vi "test14-MappingRelationshipByExternalRegistration_State.vi"() -> ()   [LabVIEW 2017, in "testcase-CSMStatusStateRegisterUnregister.lvclass"]
uses:
  testcase-CSMStatusStateRegisterUnregister.lvclass
  src/user.lib/_NEVSTOP/Communicable State Machine(CSM)/AdvanceAPI/CSM - Revert Arguments-Safe String.vi
  src/user.lib/_NEVSTOP/Communicable State Machine(CSM)/AdvanceAPI/CSM - Make String Arguments Safe.vi
  src/user.lib/_NEVSTOP/Communicable State Machine(CSM)/AdvanceAPI/CSM - Break Down Multiple States String.vi
  src/user.lib/_NEVSTOP/Communicable State Machine(CSM)/AdvanceAPI/CSM - Compact Multiple States.vi
  src/user.lib/_NEVSTOP/Communicable State Machine(CSM)/AdvanceAPI/CSM - Keywords.vi
  src/user.lib/_NEVSTOP/Communicable State Machine(CSM)/_Polymophic/CSM - Replace Marks in Messages.vi
  src/user.lib/_NEVSTOP/Communicable State Machine(CSM)/_Shared/Trim Single-line Text.vi
  src/user.lib/_NEVSTOP/Communicable State Machine(CSM)/Communicable State Machine.lvlib
  <vilib>/addons/_JKI Toolkits/VI Tester/TestCase.llb/TestCase.lvclass
  C:/Program Files (x86)/National Instruments/LabVIEW 2017/vi.lib/addons/_JKI Toolkits/VI Tester/TestCase.llb/TestCase.lvclass
panel:
  out "State History":string
  out "Rules 1":T1(array[cluster])
  out "Status In Registry 1":string[](array[string])
  out "Rules 2":T1(array[cluster])
  out "Status In Registry 2":string[](array[string])
  out "Loop Count":i32
  out "Error Array":errorcluster[](array[cluster])
  out "Rules 3":T1(array[cluster])
  out "Status In Registry 3":string[](array[string])
  out "Rules 4":T1(array[cluster])
  out "Status In Registry 4":string[](array[string])
  out "Loop Count 2":i32
  out "Error Array 2":errorcluster[](array[cluster])
  out "Entries After Removal":T1(array[cluster])
  out "TestCase out":refnum<class "testcase-CSMStatusStateRegisterUnregister.lvclass">
  in  "TestCase in":refnum<class "testcase-CSMStatusStateRegisterUnregister.lvclass">
  out "error out":errorcluster
  in  "error in (no error)":errorcluster
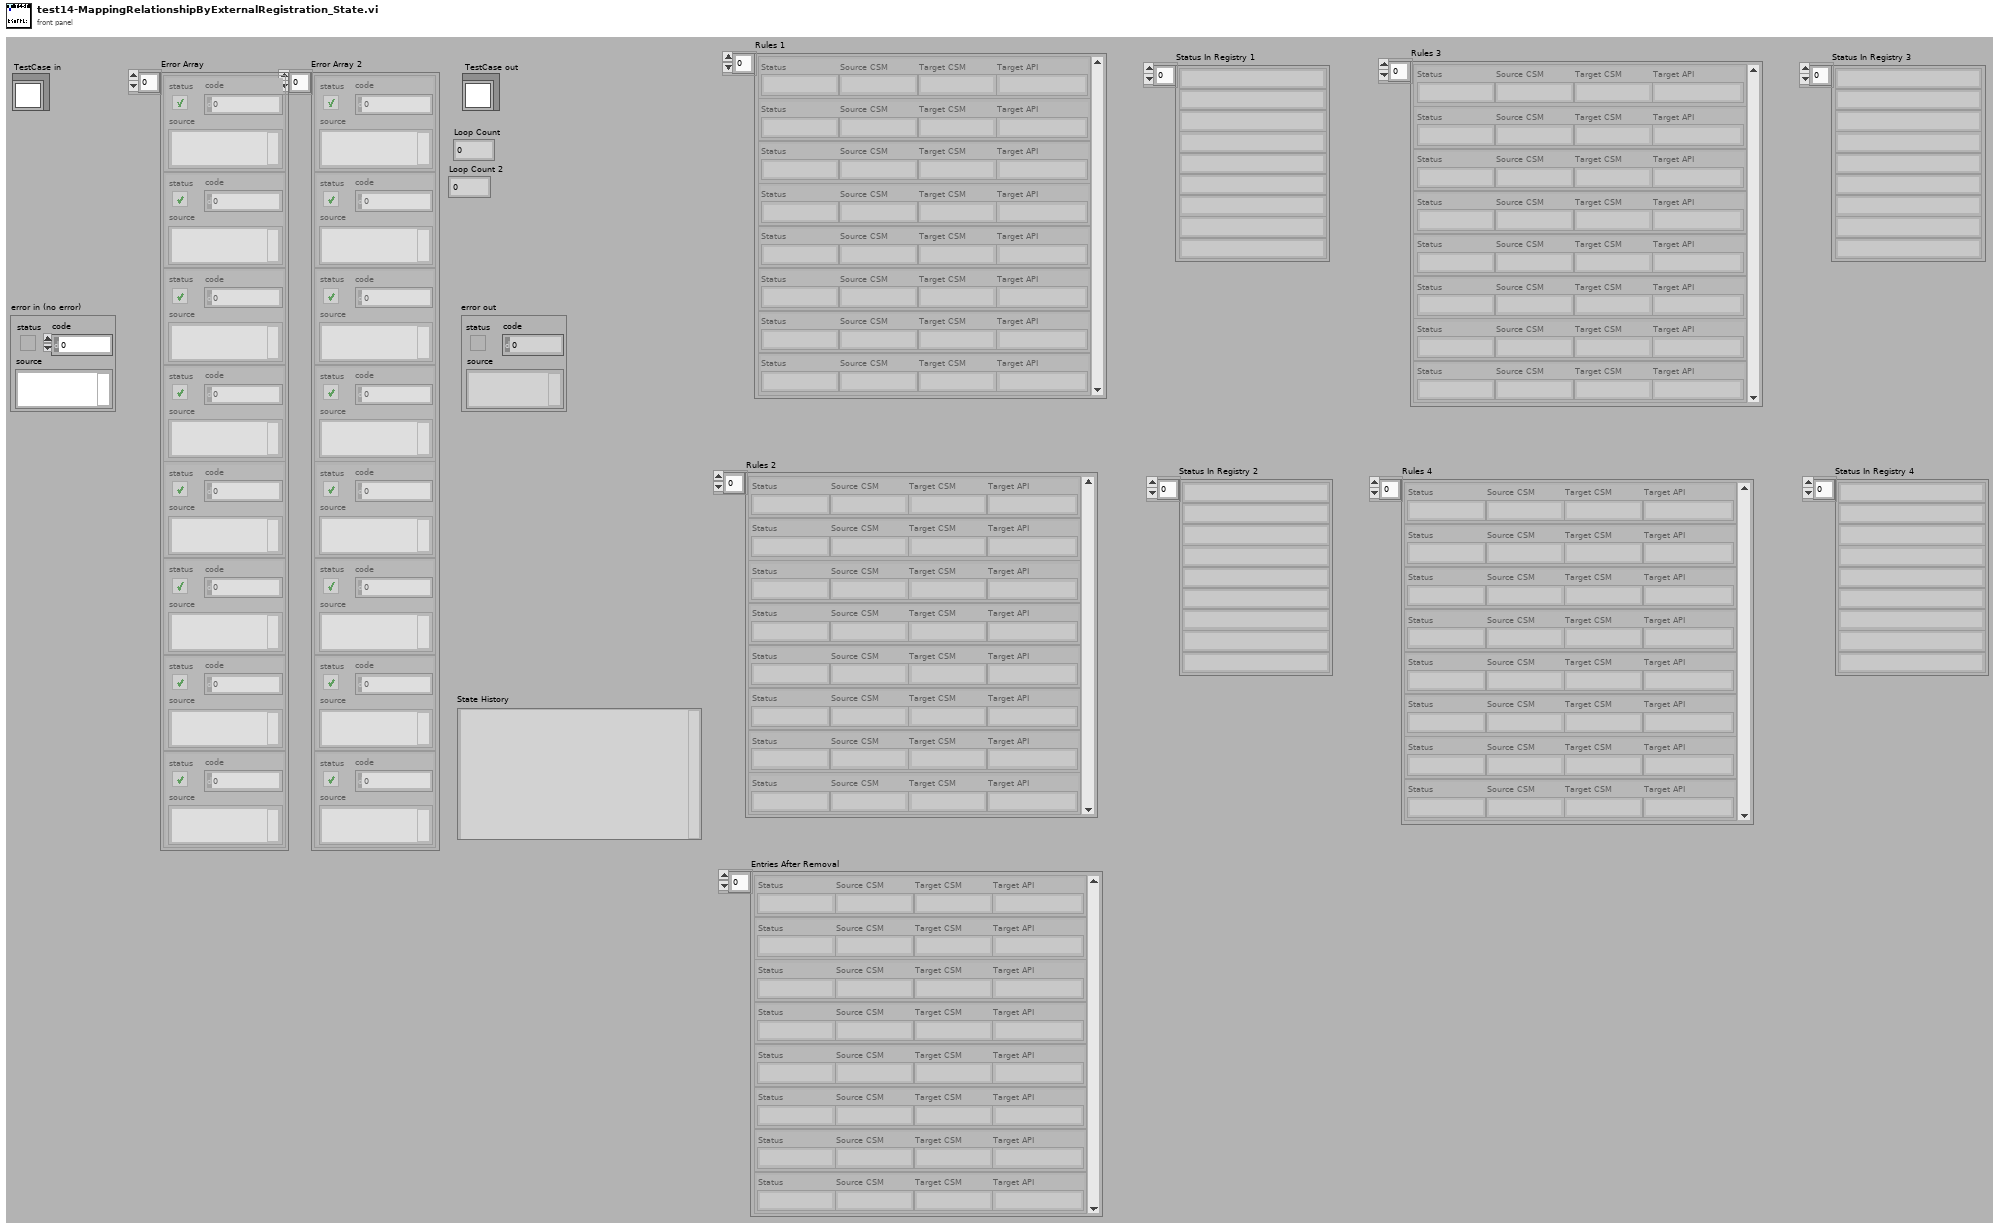
[diagram p1: front panel]
types:
  T1 = cluster{"Status":string, "Source CSM":string, "Target CSM":string, "Target API":string}[]
  T2 = enum32{"Invalid", "Standard", "Closed", "Hidden", "Minimized", "Maximized"}
  T3 = enum32{"invalid app kind", "Development System", "Run Time System", "Student Edition", "Embedded LabVIEW", "Evaluation", "Custom"}
  T4 = typedef "Communicable State Machine.lvlib/_CSM_Response Source Message.ctl" = cluster{"‘State":string, "’Arguments":string, "’Error":errorcluster}
  T5 = cluster{"Current VI Reference":refnum<vi>, "Close Panel on Exit?":bool}
  T6 = cluster{"Core":cluster{"Current VI Reference":refnum<vi>, "Close Panel on Exit?":bool}, "Your Boolean data":bool, "Your string data":string}
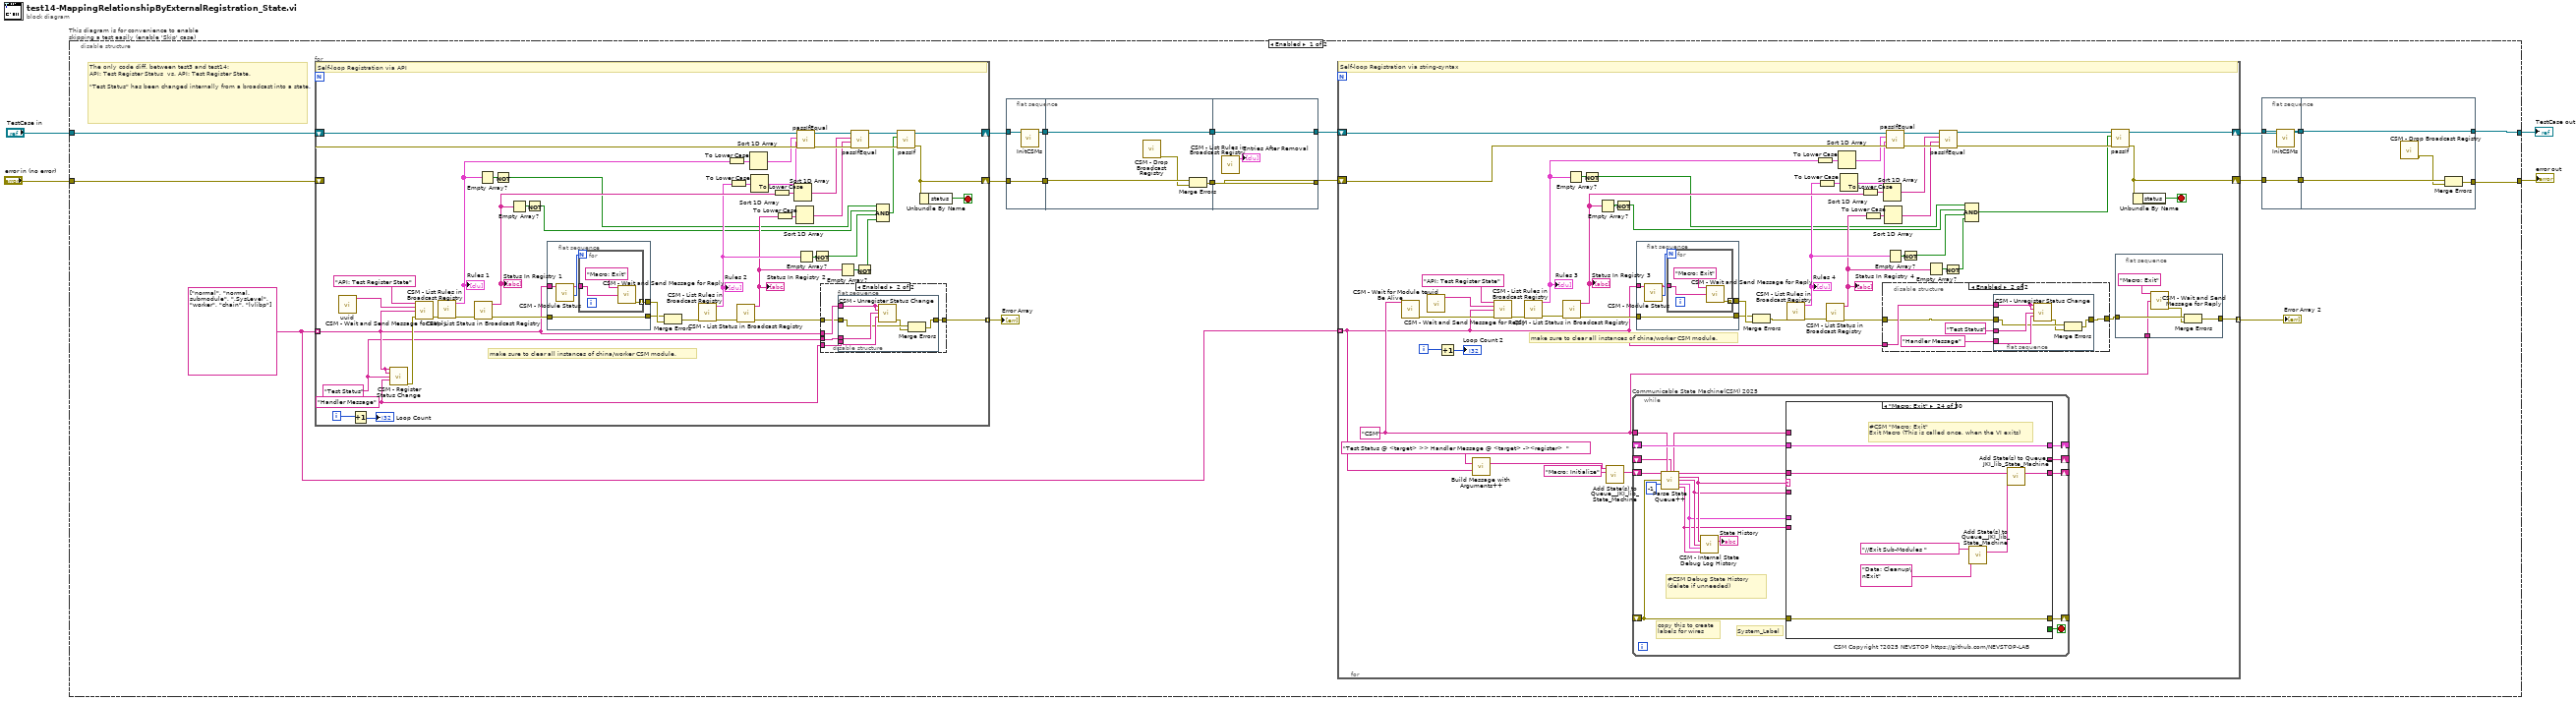
[diagram p0: block diagram]
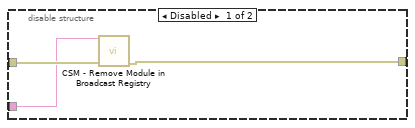
[diagram p2: hidden frame]
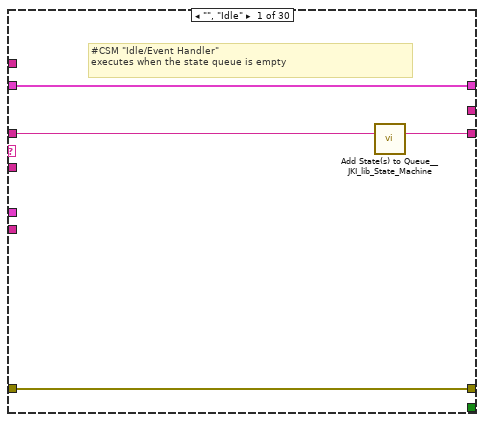
[diagram p3: hidden frame]
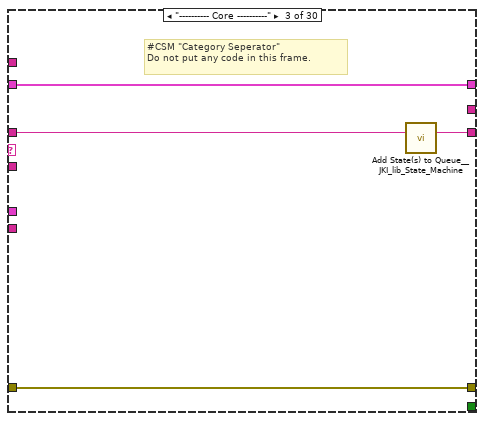
[diagram p5: hidden frame]
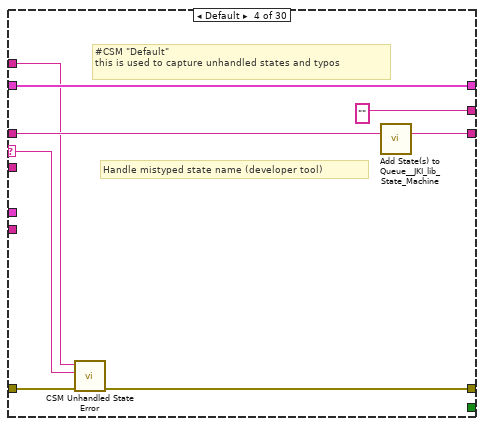
[diagram p6: hidden frame]
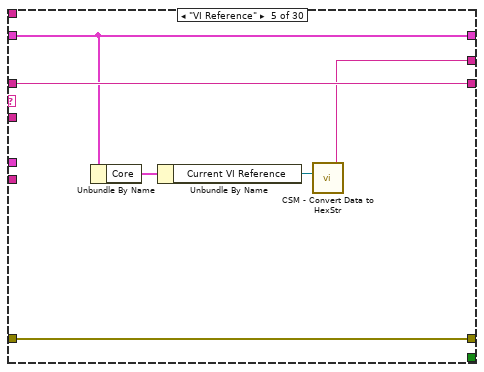
[diagram p7: hidden frame]
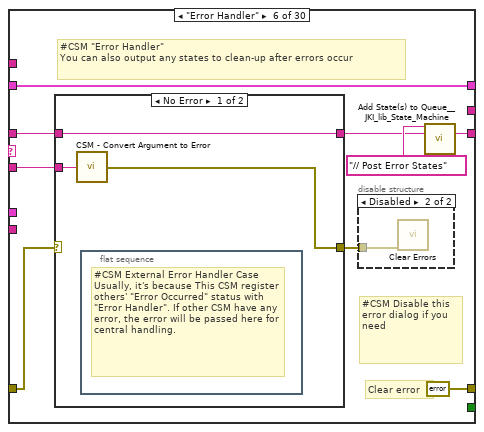
[diagram p8: hidden frame]
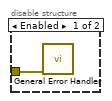
[diagram p9: hidden frame]
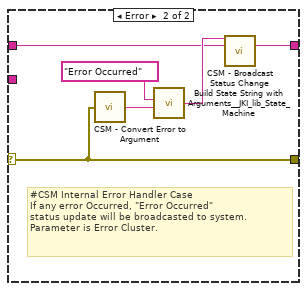
[diagram p10: hidden frame]
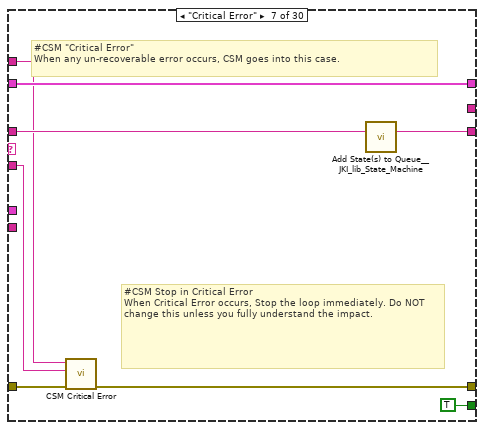
[diagram p11: hidden frame]
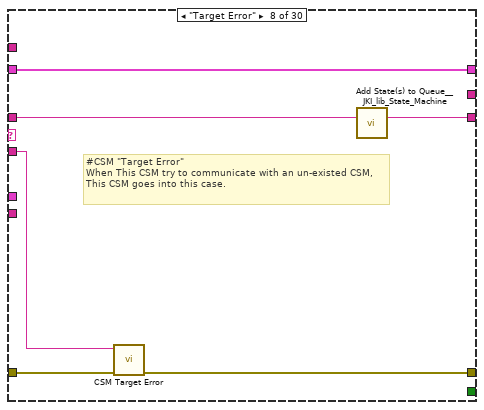
[diagram p12: hidden frame]
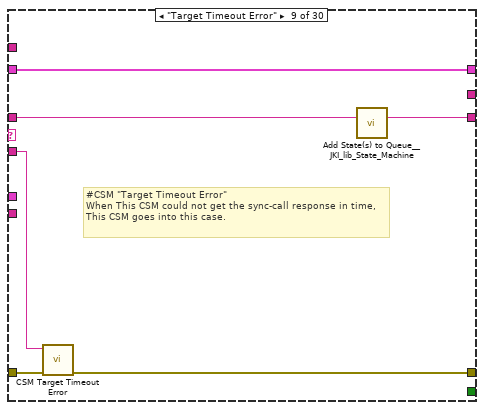
[diagram p13: hidden frame]
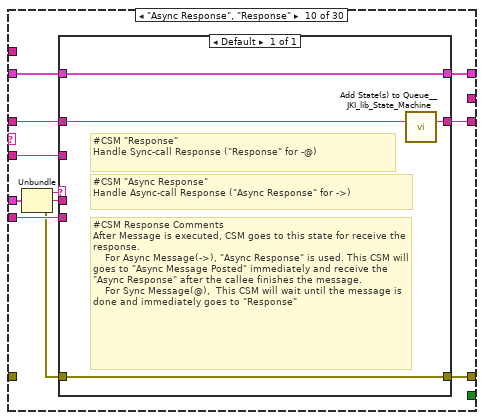
[diagram p14: hidden frame]
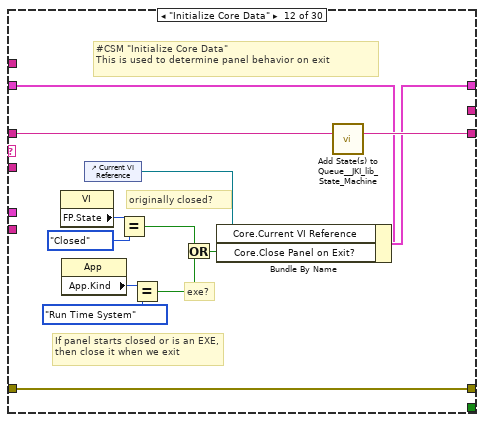
[diagram p16: hidden frame]
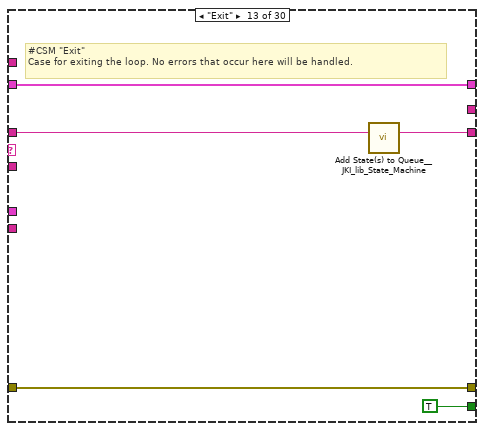
[diagram p17: hidden frame]
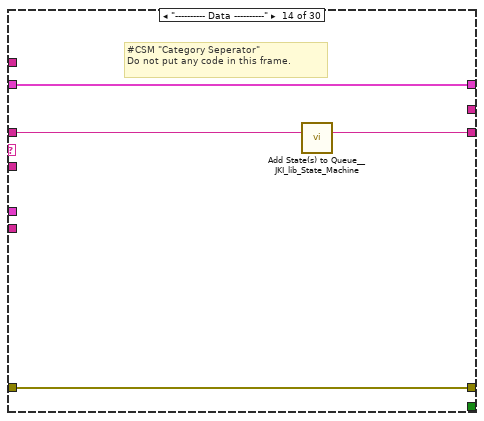
[diagram p18: hidden frame]
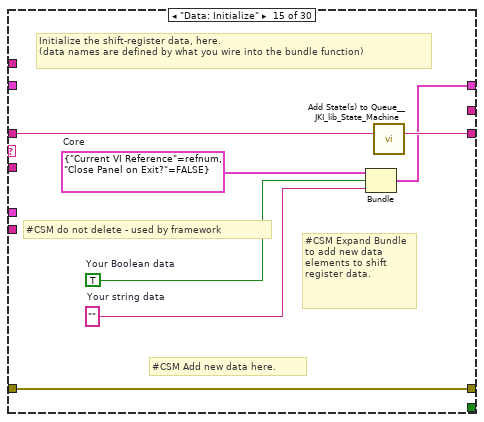
[diagram p19: hidden frame]
diagram:
  n1 = disable-structure "This diagram is for convenience to enable skipping a test easily (enable 'Skip' case)" shown="Enabled" {
    disable-tunnel: "TestCase in" -> [w23 w466]
    disable-tunnel: [w20 w464] -> w1
    disable-tunnel: [w13 w465] -> w3
    disable-tunnel: "error in (no error)" -> [w17 w463]
    frame Enabled {
      w18 = string[] ["normal", "normal.submodule", ".SysLevel", "worker", "chain", "lvlibp"]
      # "The only code diff. between test3 and test14:\nAPI: Test Register Status  vs. API: Test Register State.\n\n\"Test Status\" has been changed internally from a broadcast into a state."
      n2 = for {
        tunnel: w18 -> [w396] mode=indexing
        shift-right: [w403] -> w10
        shift-left: w23 -> [w435]
        shift-right: [w401] -> w9
        shift-left: w17 -> [w434]
        tunnel: [w397] -> w22 mode=indexing
        i -> [w420]
        stop <- w433 stop-if-true
        w395 = "Handler Message" ("Response Message (If \"\", Same as Source Message)")
        w394 = "Test Status" ("Status")
        # "make sure to clear all instances of china/worker CSM module."
        # "Self-loop Registration via API"
        n3 = call "uuid.vi"() -> ("UUID"=w439:string)  [unwired: 11 in]
        n4 = Increment(x=w420) -> (x+1=→"Loop Count":i32)
        n5 = call "CSM - Register Status Change.vi"("CSM Name"=w396, "Source CSM Name (* as Default)"=w396, "Status"=w394, "Response Message (If \"\", Same as Source Message)"=w395) -> ("error out"=w399:errorcluster)  [unwired: 10 in, 1 out]
        n6 = call "CSM - Wait and Send Message for Reply.vi"("State"="API: Test Register State", "Arguments (\"\")"=w439, "Target Module"=w396, "Error In (No Error)"=w399) -> ("error out"=w438:errorcluster)  [unwired: 9 in, 2 out]
        n7 = call "CSM - List Rules in Broadcast Registry.vi"("error in (no error)"=w438) -> ("error out"=w432:errorcluster, "Entries"=w416:T1)  [unwired: 9 in]
        "Rules 1" <- w416
        n8 = call "CSM - List Status in Broadcast Registry.vi"("error in (no error)"=w432) -> ("error out"=w418:errorcluster, "Status In Registry"=w413:string[])  [unwired: 9 in]
        "Status In Registry 1" <- w413
        n9 = Empty Array?(array=w416) -> (empty?=w415:bool)
        n10 = Not(x=w415) -> (.not. x?=w408:bool)
        n11 = Empty Array?(array=w413) -> (empty?=w414:bool)
        n12 = Not(x=w414) -> (.not. x?=w407:bool)
        n13 = flat-sequence {
          tunnel: [w459] -> w437
          tunnel: w396 -> [w457]
          tunnel: [w456] -> w417
          tunnel: w418 -> [w456]
          frame #0 {
            n14 = call "CSM - Module Status.vi"("CSM Name"=w457) -> ("#Nodes"=w458:i32, "CSM Name (Dup)"=w455:string)  [unwired: 6 in, 3 out]
            n15 = for {
              N: w458 -> [_]
              tunnel: [w461] -> w459 mode=indexing
              tunnel: w455 -> [w460]
              n16 = call "CSM - Wait and Send Message for Reply.vi"("State"="Macro: Exit", "Target Module"=w460) -> ("error out"=w461:errorcluster)  [unwired: 11 in, 2 out]
            }
          }
        }
        n17 = Merge Errors(w417, w437) -> (w436:errorcluster)
        n18 = call "CSM - List Rules in Broadcast Registry.vi"("error in (no error)"=w436) -> ("error out"=w431:errorcluster, "Entries"=w411:T1)  [unwired: 9 in]
        "Rules 2" <- w411
        n19 = To Lower Case(string=w416) -> (all lower case string=w430:T1)
        n20 = To Lower Case(string=w411) -> (all lower case string=w429:T1)
        n21 = call "CSM - List Status in Broadcast Registry.vi"("error in (no error)"=w431) -> ("error out"=w398:errorcluster, "Status In Registry"=w409:string[])  [unwired: 9 in]
        "Status In Registry 2" <- w409
        n22 = Sort 1D Array(array=w430) -> (sorted array=w428:T1)
        n23 = Sort 1D Array(array=w429) -> (sorted array=w427:T1)
        n24 = To Lower Case(string=w413) -> (all lower case string=w424:string[])
        n25 = To Lower Case(string=w409) -> (all lower case string=w423:string[])
        n26 = Sort 1D Array(array=w424) -> (sorted array=w422:string[])
        n27 = Sort 1D Array(array=w423) -> (sorted array=w421:string[])
        n28 = call-dynamic "passIfEqual.vi"("error in (no error)"=w434, "y"=w427, "x"=w428, "TestCase in"=w435) -> ("error out"=w425:errorcluster, "TestCase out"=w426:refnum<class "testcase-CSMStatusStateRegisterUnregister.lvclass">)  [unwired: 6 in]
        n29 = Empty Array?(array=w411) -> (empty?=w412:bool)
        n30 = Not(x=w412) -> (.not. x?=w406:bool)
        n31 = disable-structure shown="Enabled" {
          disable-tunnel: w398 -> [w443 w445]
          disable-tunnel: [w442 w444] -> w397
          disable-tunnel: w396 -> [w441 w446]
          disable-tunnel: w394 -> [_ w448]
          disable-tunnel: w395 -> [_ w447]
          frame Disabled {
            n32 = call "CSM - Remove Module in Broadcast Registry.vi"("CSM Name"=w441, "Error In"=w443) -> ("error out"=w442:errorcluster)  [unwired: 12 in, 1 out]
          }
          frame Enabled {
            n33 = flat-sequence {
              tunnel: w448 -> [w454]
              tunnel: w447 -> [w453]
              tunnel: w446 -> [w452]
              tunnel: w445 -> [w451]
              tunnel: [w449] -> w444
              frame #0 {
                n34 = call "CSM - Unregister Status Change.vi"("CSM Name"=w452, "Source CSM Name (* as Default)"=w452, "Status"=w454, "Response Message (\"*\" as Default)"=w453) -> ("error out"=w450:errorcluster)  [unwired: 10 in, 1 out]
                n35 = Merge Errors(w451, w450) -> (w449:errorcluster)
              }
            }
          }
        }
        n36 = Empty Array?(array=w409) -> (empty?=w410:bool)
        n37 = call-dynamic "passIfEqual.vi"("error in (no error)"=w425, "y"=w421, "x"=w422, "TestCase in"=w426) -> ("error out"=w402:errorcluster, "TestCase out"=w404:refnum<class "testcase-CSMStatusStateRegisterUnregister.lvclass">)  [unwired: 6 in]
        n38 = Not(x=w410) -> (.not. x?=w405:bool)
        n39 = Compound Arithmetic op=AND(w408, w407, w406, w405) -> (w400:bool)
        n40 = call-dynamic "passIf.vi"("error in (no error)"=w402, "pass"=w400, "TestCase in"=w404) -> ("error out"=w401:errorcluster, "TestCase out"=w403:refnum<class "testcase-CSMStatusStateRegisterUnregister.lvclass">)  [unwired: 7 in]
        n41 = Unbundle By Name(w401) -> ("status"=w433:bool)
      }
      "Error Array" <- w22
      n42 = flat-sequence {
        tunnel: w10 -> [w26]
        tunnel: [w25] -> w12
        tunnel: [w24] -> w11
        tunnel: w9 -> [w24]
        tunnel: w12 -> [w30]
        tunnel: w11 -> [w29]
        tunnel: [w30] -> w6
        tunnel: [w28] -> w5
        tunnel: [w32] -> w7
        tunnel: [w33] -> w8
        tunnel: w6 -> [w33]
        tunnel: w5 -> [w32]
        frame #0 {
          n43 = call "InitCSMs.vi"("testcase-CSMStatus in"=w26) -> ("testcase-CSMStatus out"=w25:refnum<class "testcase-CSMStatusStateRegisterUnregister.lvclass">)  [unwired: 9 in, 1 out]
        }
        frame #1 {
          n44 = call "CSM - Drop Broadcast Registry.vi"() -> ("error out"=w27:errorcluster)  [unwired: 15 in]
          n45 = Merge Errors(w29, w27) -> (w28:errorcluster)
        }
        frame #2 {
          n46 = call "CSM - List Rules in Broadcast Registry.vi"() -> ("Entries"=→"Entries After Removal":T1)  [unwired: 10 in, 1 out]
        }
      }
      n47 = for {
        tunnel: w18 -> [w41] mode=indexing
        shift-right: [w56] -> w21
        shift-left: w8 -> [w86]
        shift-right: [w54] -> w14
        shift-left: w7 -> [w85]
        tunnel: [w49] -> w19 mode=indexing
        i -> [w71]
        stop <- w84 stop-if-true
        w48 = "CSM" ("Name (\"\" to Use UUID)")
        # "make sure to clear all instances of china/worker CSM module."
        # "Self-loop Registration via string-syntax"
        n48 = call "CSM - Wait for Module to Be Alive.vi"("CSM Name"=w48) -> ("error out"=w47:errorcluster)  [unwired: 12 in, 2 out]
        n49 = call "uuid.vi"() -> ("UUID"=w90:string)  [unwired: 11 in]
        n50 = Increment(x=w71) -> (x+1=→"Loop Count 2":i32)
        n51 = call-poly "Build Message with Arguments++.vi"("States With Replace Token"="Test Status @ <target> >> Handler Message @ <target> -><register>  " ("State"), "<target>"=w41) -> ("States"=w44:string)  [unwired: 13 in]
        n52 = call "CSM - Wait and Send Message for Reply.vi"("State"="API: Test Register State", "Arguments (\"\")"=w90, "Target Module"=w41, "Error In (No Error)"=w47) -> ("error out"=w89:errorcluster)  [unwired: 9 in, 2 out]
        n53 = call "CSM - List Rules in Broadcast Registry.vi"("error in (no error)"=w89) -> ("error out"=w83:errorcluster, "Entries"=w67:T1)  [unwired: 9 in]
        "Rules 3" <- w67
        n54 = call "CSM - List Status in Broadcast Registry.vi"("error in (no error)"=w83) -> ("error out"=w69:errorcluster, "Status In Registry"=w64:string[])  [unwired: 9 in]
        "Status In Registry 3" <- w64
        n55 = Empty Array?(array=w67) -> (empty?=w66:bool)
        n56 = Not(x=w66) -> (.not. x?=w59:bool)
        n57 = Empty Array?(array=w64) -> (empty?=w65:bool)
        n58 = call <vilib>:"Add State(s) to Queue__JKI_lib_State_Machine.vi"("State(s) in Front (\"\")"=w44, "State(s) in (\"\")"="Macro: Initialize" ("Init State(\"Macro: Initialize\")")) -> ("States Out"=w45:string)  [unwired: 13 in]
        n59 = Not(x=w65) -> (.not. x?=w58:bool)
        n60 = while "Communicable State Machine(CSM) 2025" {
          shift-right: [w123] -> _
          shift-left: _ -> [w122]
          shift-right: [w126] -> _
          shift-left: _ -> [w121]
          shift-right: [w125] -> _
          shift-left: w45 -> [w127]
          tunnel: w48 -> [w119]
          shift-right: [w120] -> _
          shift-left: _ -> [w113]
          stop <- w124 stop-if-true
          # "#CSM Debug State History\n(delete if unneeded)"
          # "copy this to create labels for wires"
          # "System_Label"
          # "CSM Copyright ?2025 NEVSTOP https://github.com/NEVSTOP-LAB"
          n61 = call "Parse State Queue++.vi"("State Queue"=w127, "Name (\"\" to Use UUID)"=w119, "Response Arguments"=w113, "Previous Error"=w121, "Dequeue (1 ms)"=-1 ("Timeout")) -> ("Name Used"=w114:string, "Remaining States"=w128:string, "Current State"=w118:string, "Arguments"=w117:string, "Additional Information"=w116:T4, "Source CSM"=w115:string)  [unwired: 5 in]
          n62 = call "CSM - Internal State Debug Log History.vi"("State"=w118, "Arguments (\"\")"=w117, ">> Response Source Message >>"=w116, "Source (\"\")"=w115) -> ("Debug Log"=→"State History":string)  [unwired: 11 in]
          n63 = case shown="\"Macro: Exit\"" w118 {
            selector: w118 -> [_ _ _ w142 _ _ _ _ _ _ _ _ _ _ _ _ _ _ _ _ _ _ _ _ _ _ _ _ _ _]
            tunnel: w128 -> [w129 w134 w139 w146 w152 w158 w179 w185 w191 w199 w210 w224 w229 w233 w240 w242 w249 w253 w257 w263 w278 w347 w352 w359 w361 w365 w370 w377 w381 w385]
            tunnel: w117 -> [_ _ _ _ _ w157 w175 w184 w189 w198 _ _ _ _ _ _ _ _ _ w258 w272 _ _ _ _ _ w368 _ _ _]
            tunnel: w122 -> [w130 w133 w136 w144 w151 w161 w180 w186 w192 w201 w209 w217 w227 w230 _ w241 w244 w250 w255 w261 w274 w344 w349 w356 w360 w364 w369 w374 w378 w382]
            tunnel: [w131 w135 w137 w140 w153 errorcluster {"status"=FALSE, "code"=0, "source"=""} ("error out") w176 w182 w188 w204 w211 w221 w226 w231 w237 w243 w245 w251 w254 w259 w275 w345 w350 w357 w362 w366 w371 w375 w379 w383] -> w126
            tunnel: w121 -> [w131 w135 w137 w147 w153 w159 w181 w183 w190 _ w211 w221 w226 w231 w237 w243 w246 w251 w254 w260 w276 w345 w350 w357 w362 w366 w371 w375 w379 w383]
            tunnel: [w132 w134 w138 w145 w152 w154 w178 w187 w193 w200 w210 w223 w228 w232 w239 w242 w248 w252 w256 w262 w277 w346 w351 w358 w361 w365 w370 w376 w380 w384] -> w125
            tunnel: [_ _ _ _ _ _ TRUE _ _ _ _ _ TRUE _ _ _ _ _ _ _ _ _ _ _ _ _ _ _ _ _] -> w124
            tunnel: [w130 w133 w136 w144 w151 w161 w180 w186 w192 w202 w209 w222 w227 w230 w238 w241 w244 w250 w255 w261 w274 w344 w349 w356 w360 w364 w369 w374 w378 w382] -> w123
            tunnel: w115 -> [_ _ _ _ _ _ _ _ _ w196 _ _ _ _ _ _ _ _ _ _ _ _ _ _ _ _ _ _ _ _]
            tunnel: w116 -> [_ _ _ _ _ _ _ _ _ w203 _ _ _ _ _ _ _ _ _ _ _ _ _ _ _ _ _ _ _ _]
            tunnel: [_ _ _ "" w148 _ _ _ _ _ _ _ _ _ _ _ _ _ _ _ _ _ _ _ _ "API1 Response" w367 _ _ _] -> w120
            tunnel: w114 -> [_ _ _ w141 _ _ w174 _ _ _ _ _ _ _ _ _ _ _ _ _ _ _ _ _ _ _ _ _ _ _]
            frame "", "Idle" {
              # "#CSM \"Idle/Event Handler\"\nexecutes when the state queue is empty"
              n64 = call <vilib>:"Add State(s) to Queue__JKI_lib_State_Machine.vi"("State(s) in (\"\")"=w129) -> ("States Out"=w132:string)  [unwired: 14 in]
            }
            frame "CSM Documentation" {
              # "#CSM README FIRST\n\nCommunicable State Machine(CSM) is a LabVIEW application framework that builds upon JKI State Machine(JKISM). It follows the pattern of JKISM and extends the keywords to describe message communication between modules, including concepts such as Sync-Message, Async-Message, Subscription/Unsubscription of status - essential elements for creating reusable code modules. For more information, please visit the CSM wiki: https://nevstop-lab.github.io/CSM-Wiki/\n\nFor instructions on JKI State Machine, visit: http://jki.net/state-machine/\nFor information about CSM, visit: https://github.com/NEVSTOP-LAB"
              # "#CSM \"Documentation\"\nCase for holding CSM Documenation"
            }
            frame "---------- Core ----------" {
              # "#CSM \"Category Seperator\"\nDo not put any code in this frame."
              n65 = call <vilib>:"Add State(s) to Queue__JKI_lib_State_Machine.vi"("State(s) in (\"\")"=w139) -> ("States Out"=w138:string)  [unwired: 14 in]
            }
            frame Default {
              # "#CSM \"Default\"\nthis is used to capture unhandled states and typos"
              # "Handle mistyped state name (developer tool)"
              n66 = call "CSM Unhandled State Error.vi"("error in (no error)"=w147, "Undefined State"=w142, "CSM Name"=w141) -> ("error out"=w140:errorcluster)  [unwired: 8 in]
              n67 = call <vilib>:"Add State(s) to Queue__JKI_lib_State_Machine.vi"("State(s) in (\"\")"=w146) -> ("States Out"=w145:string)  [unwired: 14 in]
            }
            frame "VI Reference" {
              n68 = Unbundle By Name(w151) -> ("Core"=w150:T5)
              n69 = Unbundle By Name(w150) -> ("Current VI Reference"=w149:refnum<vi>)
              n70 = call "CSM - Convert Data to HexStr.vi"("Variant"=w149) -> ("HEX String (0-9,A-F)"=w148:string)  [unwired: 8 in]
            }
            frame "Error Handler" {
              # "#CSM Disable this error dialog if you need"
              # "#CSM \"Error Handler\"\nYou can also output any states to clean-up after errors occur"
              # "Clear error"
              n71 = case shown="No Error" w159 {
                selector: w159 -> [_ w168]
                tunnel: [w167 w170] -> w155
                tunnel: w158 -> [w167 w169]
                tunnel: w157 -> [w166 _]
                tunnel: [w165 w168] -> w160
                frame No Error {
                  n72 = call "CSM - Convert Argument to Error.vi"("Argument"=w166) -> ("Error"=w165:errorcluster)  [unwired: 4 in]
                  n73 = flat-sequence {
                    frame #0 {
                      # "#CSM External Error Handler Case\nUsually, it's because This CSM register others' \"Error Occurred\" status with \"Error Handler\". If other CSM have any error, the error will be passed here for central handling."
                    }
                  }
                }
                frame Error {
                  # "#CSM Internal Error Handler Case \nIf any error Occurred, \"Error Occurred\" \nstatus update will be broadcasted to system.\nParameter is Error Cluster."
                  n74 = call "CSM - Convert Error to Argument.vi"("Error"=w168) -> ("Argument"=w172:string)  [unwired: 4 in]
                  n75 = call <vilib>:"Build State String with Arguments__JKI_lib_State_Machine.vi"("Arguments (\"\")"=w172, "State"="Error Occurred" ("Status with Arguments")) -> ("State with Arguments"=w171:string)  [unwired: 4 in]
                  n76 = call "CSM - Broadcast Status Change.vi"("Status With Arguments"=w171, "State Queue"=w169) -> ("Remaining States"=w170:string)  [unwired: 13 in]
                }
              }
              n77 = disable-structure shown="Disabled" {
                disable-tunnel: w160 -> [w163 w164]
                frame Enabled {
                  n78 = call <vilib>:"General Error Handler.vi"("error in (no error)"=w163) -> ()  [unwired: 10 in, 5 out]
                }
                frame Disabled {
                  n79 = call <vilib>:"Clear Errors.vi"("error in (no error)"=w164) -> ()  [unwired: 5 in, 2 out]
                }
              }
              n80 = call <vilib>:"Add State(s) to Queue__JKI_lib_State_Machine.vi"("State(s) in Front (\"\")"="// Post Error States", "State(s) in (\"\")"=w155) -> ("States Out"=w154:string)  [unwired: 13 in]
            }
            frame "Critical Error" {
              # "#CSM Stop in Critical Error\nWhen Critical Error occurs, Stop the loop immediately. Do NOT change this unless you fully understand the impact."
              # "#CSM \"Critical Error\"\nWhen any un-recoverable error occurs, CSM goes into this case."
              n81 = call "CSM Critical Error.vi"("error in (no error)"=w181, "Arugments (As Reason)"=w175, "CSM Name"=w174) -> ("error out"=w176:errorcluster)  [unwired: 8 in]
              n82 = call <vilib>:"Add State(s) to Queue__JKI_lib_State_Machine.vi"("State(s) in (\"\")"=w179) -> ("States Out"=w178:string)  [unwired: 14 in]
            }
            frame "Target Error" {
              # "#CSM \"Target Error\"\nWhen This CSM try to communicate with an un-existed CSM, This CSM goes into this case."
              n83 = call "CSM Target Error.vi"("error in (no error)"=w183, "Arguments (As CSM Name)"=w184) -> ("error out"=w182:errorcluster)  [unwired: 9 in]
              n84 = call <vilib>:"Add State(s) to Queue__JKI_lib_State_Machine.vi"("State(s) in (\"\")"=w185) -> ("States Out"=w187:string)  [unwired: 14 in]
            }
            frame "Target Timeout Error" {
              # "#CSM \"Target Timeout Error\"\nWhen This CSM could not get the sync-call response in time, This CSM goes into this case."
              n85 = call "CSM Target Timeout Error.vi"("error in (no error)"=w190, "Arguments (As CSM Name)"=w189) -> ("error out"=w188:errorcluster)  [unwired: 9 in]
              n86 = call <vilib>:"Add State(s) to Queue__JKI_lib_State_Machine.vi"("State(s) in (\"\")"=w191) -> ("States Out"=w193:string)  [unwired: 14 in]
            }
            frame "Async Response", "Response" {
              n87 = Unbundle(w203) -> ("‘State"=w197:string, "’Arguments"=w195:string, "’Error"=w194:errorcluster)
              n88 = case shown="Default" w197 {
                tunnel: [w208] -> w204
                tunnel: w194 -> [w208]
                tunnel: [w207] -> w202
                tunnel: w201 -> [w207]
                tunnel: [w205] -> w200
                tunnel: w199 -> [w206]
                tunnel: w198 -> [_]
                tunnel: w196 -> [_]
                tunnel: w195 -> [_]
                frame Default {
                  # "#CSM Response Comments\nAfter Message is executed, CSM goes to this state for receive the response.\n    For Async Message(->), \"Async Response\" is used. This CSM will goes to \"Async Message Posted\" immediately and receive the \"Async Response\" after the callee finishes the message.\n    For Sync Message(@),  This CSM will wait until the message is done and immediately goes to \"Response\""
                  # "#CSM \"Async Response\"\nHandle Async-call Response (\"Async Response\" for ->)"
                  # "#CSM \"Response\"\nHandle Sync-call Response (\"Response\" for -@)"
                  n89 = call <vilib>:"Add State(s) to Queue__JKI_lib_State_Machine.vi"("State(s) in (\"\")"=w206) -> ("States Out"=w205:string)  [unwired: 14 in]
                }
              }
            }
            frame "Async Message Posted" {
              # "#CSM \"Async Message Posted\"\nAfter Async Message is posted (-> or ->| ), CSM goes to this state for post-action.\nYou can use Argument - State to tell which Async Message is called."
            }
            frame "Initialize Core Data" {
              # "#CSM \"Initialize Core Data\"\nThis is used to determine panel behavior on exit"
              # "originally closed?"
              # "exe?"
              # "If panel starts closed or is an EXE, then close it when we exit"
              n90 = property class="VI"() -> ("FP.State"=w214:T2)  [unwired: 2 in, 2 out]
              n91 = property class="App"() -> ("App.Kind"=w220:T3)  [unwired: 2 in, 2 out]
              n92 = control-ref of="Current VI Reference"() -> (w215:refnum<vi>)
              n93 = Equal?(x=w214, y=T2."Closed" ("Front Panel Window:State")) -> (x = y?=w212:bool)
              n94 = Equal?(x=w220, y=T3."Run Time System" ("Application:Kind")) -> (x = y?=w218:bool)
              n95 = Or(x=w212, y=w218) -> (x .or. y?=w216:bool)
              n96 = Bundle By Name(cluster=w217, "Core.Current VI Reference"=w215, "Core.Close Panel on Exit?"=w216) -> (w222:T6)
              n97 = call <vilib>:"Add State(s) to Queue__JKI_lib_State_Machine.vi"("State(s) in (\"\")"=w224) -> ("States Out"=w223:string)  [unwired: 14 in]
            }
            frame "Exit" {
              # "#CSM \"Exit\"\nCase for exiting the loop. No errors that occur here will be handled."
              n98 = call <vilib>:"Add State(s) to Queue__JKI_lib_State_Machine.vi"("State(s) in (\"\")"=w229) -> ("States Out"=w228:string)  [unwired: 14 in]
            }
            frame "---------- Data ----------" {
              # "#CSM \"Category Seperator\"\nDo not put any code in this frame."
              n99 = call <vilib>:"Add State(s) to Queue__JKI_lib_State_Machine.vi"("State(s) in (\"\")"=w233) -> ("States Out"=w232:string)  [unwired: 14 in]
            }
            frame "Data: Initialize" {
              w234 = T5 {"Current VI Reference"=refnum, "Close Panel on Exit?"=FALSE}  # Core
              w236 = TRUE  # Your Boolean data
              w235 = ""  # Your string data
              # "#CSM do not delete - used by framework"
              # "#CSM Expand Bundle to add new data elements to shift register data."
              # "#CSM Add new data here."
              # "Initialize the shift-register data, here.\n(data names are defined by what you wire into the bundle function)"
              n100 = Bundle("Core"=w234, "Your Boolean data"=w236, "Your string data"=w235) -> (w238:T6)  [unwired: 1 in]
              n101 = call <vilib>:"Add State(s) to Queue__JKI_lib_State_Machine.vi"("State(s) in (\"\")"=w240) -> ("States Out"=w239:string)  [unwired: 14 in]
            }
            frame "Data: Update Indicators" {
            }
            frame "Data: Cleanup" {
              # "Cleanup any data and references, here.\n(this is called automatically, by the Macro: Exit)"
              n102 = Unbundle By Name(w244) -> ("Core.Current VI Reference"=w247:refnum<vi>)
              n103 = Close Reference(reference=w247, error in (no error)=w246) -> (error out=w245:errorcluster)
              n104 = call <vilib>:"Add State(s) to Queue__JKI_lib_State_Machine.vi"("State(s) in (\"\")"=w249) -> ("States Out"=w248:string)  [unwired: 14 in]
            }
            frame "---------- UI ----------" {
              # "#CSM \"Category Seperator\"\nDo not put any code in this frame."
              n105 = call <vilib>:"Add State(s) to Queue__JKI_lib_State_Machine.vi"("State(s) in (\"\")"=w253) -> ("States Out"=w252:string)  [unwired: 14 in]
            }
            frame "UI: Initialize" {
              # "#CSM \"UI: Initialize\"\nInitialize the User Interface, here.\n(this is called automatically, by the Macro: Init)"
              n106 = call <vilib>:"Add State(s) to Queue__JKI_lib_State_Machine.vi"("State(s) in (\"\")"=w257) -> ("States Out"=w256:string)  [unwired: 14 in]
            }
            frame "UI: Cursor Set" {
              # "#CSM \"UI: Cursor Set\"\nSet and Unset Cursor Busy.\n(Usage: \"UI: Cursor Set >> Busy|Idle\")"
              # "Argument"
              n107 = disable-structure shown="TARGET_TYPE!=Windows" {
                disable-tunnel: w260 -> [w266 w271]
                disable-tunnel: [w265 w271] -> w259
                disable-tunnel: w258 -> [w264 _]
                frame condition #0 (active) {
                  n108 = case shown="\"Idle\", Default" w264 {
                    tunnel: w266 -> [w268 w270]
                    tunnel: [w267 w269] -> w265
                    frame "Idle", Default {
                      n109 = call <vilib>:"Unset Busy.vi"("error in (no error)"=w268) -> ("error out"=w267:errorcluster)  [unwired: 10 in]
                    }
                    frame "Busy" {
                      n110 = call <vilib>:"Set Busy.vi"("error in (no error)"=w270) -> ("error out"=w269:errorcluster)  [unwired: 9 in, 1 out]
                    }
                  }
                }
                frame condition #1 {
                }
              }
              n111 = call <vilib>:"Add State(s) to Queue__JKI_lib_State_Machine.vi"("State(s) in (\"\")"=w263) -> ("States Out"=w262:string)  [unwired: 14 in]
            }
            frame "UI: Front Panel State" {
              # "#CSM \"UI: Front Panel State\"\nSet Front Panel Open or Closed\n(Usage: \"UI: Front Panel State >> Open|Close\")"
              # "Argument"
              n112 = Unbundle By Name(w274) -> ("Core.Current VI Reference"=w273:refnum<vi>)
              n113 = call <vilib>:"Add State(s) to Queue__JKI_lib_State_Machine.vi"("State(s) in (\"\")"=w278) -> ("States Out"=w277:string)  [unwired: 14 in]
              n114 = case shown="\"Close\", \"Closed\"" w272 {
                tunnel: w276 -> [w284 w299 w310 w323 w336]
                tunnel: [w286 w300 w312 w325 w338] -> w275
                tunnel: w273 -> [w285 w297 w311 w324 w337]
                frame "Open", "Standard", Default {
                  w279 = T2."Standard" ("State")
                  n115 = property class="VI"(reference=w285, error in=w284) -> (reference out=w282:refnum<vi>, error out=w283:errorcluster, "FP.State"=w281:T2)
                  n116 = Not Equal?(x=w281, y=w279) -> (x != y?=w280:bool)
                  n117 = case shown="True" w280 {
                    tunnel: [w290 w292] -> w286
                    tunnel: w283 -> [w289 w292]
                    tunnel: w282 -> [w288 _]
                    tunnel: w279 -> [w287 _]
                    frame True {
                      n118 = invoke class="VI" method="FP.Open"(reference=w288, error in=w289, "Activate"=TRUE, "State"=w287) -> (error out=w290:errorcluster)  [unwired: 1 in, 4 out]
                    }
                    frame False {
                    }
                  }
                }
                frame "Close", "Closed" {
                  n119 = property class="VI"(reference=w297, error in=w299) -> (reference out=w296:refnum<vi>, error out=w298:errorcluster, "FP.State"=w294:T2)
                  n120 = Not Equal?(x=w294, y=T2."Closed" ("Front Panel Window:State")) -> (x != y?=w293:bool)
                  n121 = case shown="False" w293 {
                    tunnel: [w301 w304] -> w300
                    tunnel: w298 -> [w301 w303]
                    tunnel: w296 -> [_ w302]
                    frame False {
                    }
                    frame True {
                      n122 = invoke class="VI" method="FP.Close"(reference=w302, error in=w303) -> (error out=w304:errorcluster)  [unwired: 1 in, 2 out]
                    }
                  }
                }
                frame "Hidden", "Hide" {
                  w305 = T2."Hidden" ("State")
                  n123 = property class="VI"(reference=w311, error in=w310) -> (reference out=w308:refnum<vi>, error out=w309:errorcluster, "FP.State"=w307:T2)
                  n124 = Not Equal?(x=w307, y=w305) -> (x != y?=w306:bool)
                  n125 = case shown="True" w306 {
                    tunnel: [w316 w317] -> w312
                    tunnel: w309 -> [w315 w317]
                    tunnel: w308 -> [w314 _]
                    tunnel: w305 -> [w313 _]
                    frame True {
                      n126 = invoke class="VI" method="FP.Open"(reference=w314, error in=w315, "State"=w313) -> (error out=w316:errorcluster)  [unwired: 2 in, 4 out]
                    }
                    frame False {
                    }
                  }
                }
                frame "Minimize", "Minimized" {
                  w318 = T2."Minimized" ("State")
                  n127 = property class="VI"(reference=w324, error in=w323) -> (reference out=w321:refnum<vi>, error out=w322:errorcluster, "FP.State"=w320:T2)
                  n128 = Not Equal?(x=w320, y=w318) -> (x != y?=w319:bool)
                  n129 = case shown="True" w319 {
                    tunnel: [w329 w330] -> w325
                    tunnel: w322 -> [w328 w330]
                    tunnel: w321 -> [w327 _]
                    tunnel: w318 -> [w326 _]
                    frame True {
                      n130 = invoke class="VI" method="FP.Open"(reference=w327, error in=w328, "State"=w326) -> (error out=w329:errorcluster)  [unwired: 2 in, 4 out]
                    }
                    frame False {
                    }
                  }
                }
                frame "Maximize", "Maximized" {
                  w331 = T2."Maximized" ("State")
                  n131 = property class="VI"(reference=w337, error in=w336) -> (reference out=w334:refnum<vi>, error out=w335:errorcluster, "FP.State"=w333:T2)
                  n132 = Not Equal?(x=w333, y=w331) -> (x != y?=w332:bool)
                  n133 = case shown="True" w332 {
                    tunnel: [w342 w343] -> w338
                    tunnel: w335 -> [w341 w343]
                    tunnel: w334 -> [w340 _]
                    tunnel: w331 -> [w339 _]
                    frame True {
                      n134 = invoke class="VI" method="FP.Open"(reference=w340, error in=w341, "State"=w339) -> (error out=w342:errorcluster)  [unwired: 2 in, 4 out]
                    }
                    frame False {
                    }
                  }
                }
              }
            }
            frame "---------- Macro ----------" {
              # "#CSM \"Category Seperator\"\nDo not put any code in this frame."
              n135 = call <vilib>:"Add State(s) to Queue__JKI_lib_State_Machine.vi"("State(s) in (\"\")"=w347) -> ("States Out"=w346:string)  [unwired: 14 in]
            }
            frame "Macro: Initialize" {
              # "#CSM \"Macro: Initialize\"\nInitialization Macro (This is called once, when the VI starts)"
              n136 = call <vilib>:"Add State(s) to Queue__JKI_lib_State_Machine.vi"("State(s) in Front (\"\")"="Data: Initialize\nInitialize Core Data\nData: Update Indicators", "State(s) in (\"\")"=w352) -> ("States Out"=w351:string)  [unwired: 13 in]
            }
            frame "Macro: Exit" {
              # "#CSM \"Macro: Exit\"\nExit Macro (This is called once, when the VI exits)"
              n137 = call <vilib>:"Add State(s) to Queue__JKI_lib_State_Machine.vi"("State(s) in Front (\"\")"="//Exit Sub-Modules ", "State(s) at Back (\"\")"="Data: Cleanup\nExit") -> ("States Out"=w354:string)  [unwired: 13 in]
              n138 = call <vilib>:"Add State(s) to Queue__JKI_lib_State_Machine.vi"("State(s) in Front (\"\")"=w354, "State(s) in (\"\")"=w359) -> ("States Out"=w358:string)  [unwired: 13 in]
            }
            frame "---------- API ----------" {
              # "#CSM \"Category Seperator\"\nDo not put any code in this frame."
            }
            frame "API: API1" {
              # "#CSM API Example\nCopy/Rename this case for your own API"
              # "#CSM Response\nConnect this to return the response of your API"
              # "#CSM >> Msg/Rep's CSM >>\nIf you need to tell who triggered this state , use this string. If it's this case itself, this string is \"\"."
              # "#CSM >> Arguments >>\nDeal with the parameter if any"
            }
            frame "API: API2" {
              # "#CSM API Example\nCopy/Rename this case for your own API"
              # "unpack Hex String  to Variant\nif complex parameter is needed."
              n139 = call "CSM - Convert HexStr to Data.vi"("HEX String"=w368) -> ()  [unwired: 7 in, 2 out]
              n140 = disable-structure shown="Disabled" {
                disable-tunnel: [w372 "API2 Response"] -> w367
                frame Disabled {
                  # "pack variant to hexstr \nif complex response is needed."
                  # "complex Response"
                  n141 = call "CSM - Convert Data to HexStr.vi"() -> ("HEX String (0-9,A-F)"=w372:string)  [unwired: 9 in]
                }
                frame Enabled {
                }
              }
            }
            frame "---------- Action ----------" {
              # "#CSM \"Category Seperator\"\nDo not put any code in this frame."
              n142 = call <vilib>:"Add State(s) to Queue__JKI_lib_State_Machine.vi"("State(s) in (\"\")"=w377) -> ("States Out"=w376:string)  [unwired: 14 in]
            }
            frame "Action: action1" {
              # "#CSM \"Internal State\"\nThis category is used for holding internal states"
              n143 = call <vilib>:"Add State(s) to Queue__JKI_lib_State_Machine.vi"("State(s) in (\"\")"=w381) -> ("States Out"=w380:string)  [unwired: 14 in]
            }
            frame "Action: action2" {
              # "#CSM \"Internal State\"\nThis category is used for holding internal states"
              n144 = call <vilib>:"Add State(s) to Queue__JKI_lib_State_Machine.vi"("State(s) in (\"\")"=w385) -> ("States Out"=w384:string)  [unwired: 14 in]
            }
          }
        }
        n145 = flat-sequence {
          tunnel: [w390] -> w88
          tunnel: w41 -> [w388]
          tunnel: [w387] -> w68
          tunnel: w69 -> [w387]
          frame #0 {
            n146 = call "CSM - Module Status.vi"("CSM Name"=w388) -> ("#Nodes"=w389:i32, "CSM Name (Dup)"=w386:string)  [unwired: 6 in, 3 out]
            n147 = for {
              N: w389 -> [_]
              tunnel: [w392] -> w390 mode=indexing
              tunnel: w386 -> [w391]
              n148 = call "CSM - Wait and Send Message for Reply.vi"("State"="Macro: Exit", "Target Module"=w391) -> ("error out"=w392:errorcluster)  [unwired: 11 in, 2 out]
            }
          }
        }
        n149 = Merge Errors(w68, w88) -> (w87:errorcluster)
        n150 = call "CSM - List Rules in Broadcast Registry.vi"("error in (no error)"=w87) -> ("error out"=w82:errorcluster, "Entries"=w62:T1)  [unwired: 9 in]
        "Rules 4" <- w62
        n151 = To Lower Case(string=w67) -> (all lower case string=w81:T1)
        n152 = To Lower Case(string=w62) -> (all lower case string=w80:T1)
        n153 = call "CSM - List Status in Broadcast Registry.vi"("error in (no error)"=w82) -> ("error out"=w43:errorcluster, "Status In Registry"=w60:string[])  [unwired: 9 in]
        "Status In Registry 4" <- w60
        n154 = Sort 1D Array(array=w81) -> (sorted array=w79:T1)
        n155 = Sort 1D Array(array=w80) -> (sorted array=w78:T1)
        n156 = To Lower Case(string=w64) -> (all lower case string=w75:string[])
        n157 = To Lower Case(string=w60) -> (all lower case string=w74:string[])
        n158 = disable-structure shown="Enabled" {
          disable-tunnel: w43 -> [w94 w98]
          disable-tunnel: w41 -> [w93 w99]
          disable-tunnel: [w92 w97] -> w42
          frame Disabled {
            n159 = call "CSM - Remove Module in Broadcast Registry.vi"("CSM Name"=w93, "Error In"=w94) -> ("error out"=w92:errorcluster)  [unwired: 12 in, 1 out]
          }
          frame Enabled {
            n160 = flat-sequence {
              tunnel: "Test Status" ("Status") -> [w105]
              tunnel: "Handler Message" ("Response Message (If \"\", Same as Source Message)") -> [w104]
              tunnel: w99 -> [w103]
              tunnel: w98 -> [w102]
              tunnel: [w100] -> w97
              frame #0 {
                n161 = call "CSM - Unregister Status Change.vi"("CSM Name"=w103, "Source CSM Name (* as Default)"=w103, "Status"=w105, "Response Message (\"*\" as Default)"=w104) -> ("error out"=w101:errorcluster)  [unwired: 10 in, 1 out]
                n162 = Merge Errors(w102, w101) -> (w100:errorcluster)
              }
            }
          }
        }
        n163 = Sort 1D Array(array=w75) -> (sorted array=w73:string[])
        n164 = Sort 1D Array(array=w74) -> (sorted array=w72:string[])
        n165 = call-dynamic "passIfEqual.vi"("error in (no error)"=w85, "y"=w78, "x"=w79, "TestCase in"=w86) -> ("error out"=w76:errorcluster, "TestCase out"=w77:refnum<class "testcase-CSMStatusStateRegisterUnregister.lvclass">)  [unwired: 6 in]
        n166 = Empty Array?(array=w62) -> (empty?=w63:bool)
        n167 = Not(x=w63) -> (.not. x?=w52:bool)
        n168 = Empty Array?(array=w60) -> (empty?=w61:bool)
        n169 = call-dynamic "passIfEqual.vi"("error in (no error)"=w76, "y"=w72, "x"=w73, "TestCase in"=w77) -> ("error out"=w55:errorcluster, "TestCase out"=w57:refnum<class "testcase-CSMStatusStateRegisterUnregister.lvclass">)  [unwired: 6 in]
        n170 = Not(x=w61) -> (.not. x?=w51:bool)
        n171 = Compound Arithmetic op=AND(w59, w58, w52, w51) -> (w53:bool)
        n172 = call-dynamic "passIf.vi"("error in (no error)"=w55, "pass"=w53, "TestCase in"=w57) -> ("error out"=w54:errorcluster, "TestCase out"=w56:refnum<class "testcase-CSMStatusStateRegisterUnregister.lvclass">)  [unwired: 7 in]
        n173 = flat-sequence {
          tunnel: w42 -> [w109]
          tunnel: [w108] -> w49
          tunnel: w48 -> [w106]
          frame #0 {
            n174 = call "CSM - Wait and Send Message for Reply.vi"("State"="Macro: Exit", "Target Module"=w106) -> ("error out"=w107:errorcluster)  [unwired: 11 in, 2 out]
            n175 = Merge Errors(w109, w107) -> (w108:errorcluster)
          }
        }
        n176 = Unbundle By Name(w54) -> ("status"=w84:bool)
      }
      "Error Array 2" <- w19
      n177 = flat-sequence {
        tunnel: w21 -> [w36]
        tunnel: [w35] -> w16
        tunnel: [w34] -> w15
        tunnel: w14 -> [w34]
        tunnel: [w40] -> w20
        tunnel: w16 -> [w40]
        tunnel: w15 -> [w39]
        tunnel: [w38] -> w13
        frame #0 {
          n178 = call "InitCSMs.vi"("testcase-CSMStatus in"=w36) -> ("testcase-CSMStatus out"=w35:refnum<class "testcase-CSMStatusStateRegisterUnregister.lvclass">)  [unwired: 9 in, 1 out]
        }
        frame #1 {
          n179 = call "CSM - Drop Broadcast Registry.vi"() -> ("error out"=w37:errorcluster)  [unwired: 15 in]
          n180 = Merge Errors(w39, w37) -> (w38:errorcluster)
        }
      }
    }
    frame Disabled {
      # "skip test result while test is under development"
      n181 = call <vilib>:"skip.vi"("error in (no error)"=w463, "TestCase in"=w466) -> ("error out"=w465:errorcluster, "TestCase out"=w464:refnum<class "testcase-CSMStatusStateRegisterUnregister.lvclass">)  [unwired: 8 in]
    }
  }
  "error out" <- w3
  "TestCase out" <- w1
